vi "Teleop.vi"(10 "Match Info":T1={"Autonomous Elapsed Seconds"=0.0, "TeleOp Elapsed Seconds"=0.0, "Disabled Elapsed Seconds"=0.0, "Visited Autonomous"=FALSE, "Visited TeleOp"=FALSE, "Visited Disabled"=FALSE, "Autonomous Settings"={"Autonomous Style"=enum."Independent", "VI Refnum"=refnum}}, 11 "Call Context":T2) -> ()   [LabVIEW 2018]
doc: "This VI is called for each TeleOp packet received from the DS where the robot is not disabled. It is often used to read from the joysticks and update I/O or to update setpoints for timed control loops. It should complete and return within 20 milliseconds or it may miss DS packets."
uses:
  <vilib>/Rock Robotics/WPI/DriverStation/WPI_DriverStationDerivedRobotMode.ctl
  <vilib>/Rock Robotics/WPI/DriverStation/WPI_DriverStationMatch Info.ctl
  Functions/Global Variables/Robot State.vi
  Functions/Global Variables/Trajectory Enabled.vi
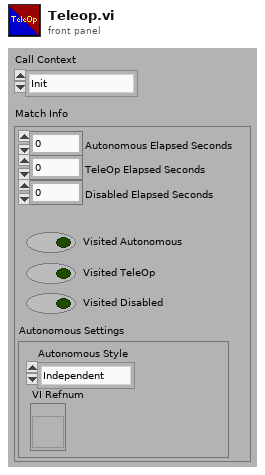
[diagram p1: front panel]
types:
  T1 = typedef "WPI_DriverStationMatch Info.ctl" = cluster{"Autonomous Elapsed Seconds":dbl, "TeleOp Elapsed Seconds":dbl, "Disabled Elapsed Seconds":dbl, "Visited Autonomous":bool, "Visited TeleOp":bool, "Visited Disabled":bool, "Autonomous Settings":cluster{"Autonomous Style":enum16{"Iterative", "Independent"}, "VI Refnum":refnum<vi>}}
  T2 = typedef "WPI_DriverStationDerivedRobotMode.ctl" = enum16{"Init", "Execute", "Stop"}
  T3 = typedef "Robot State.ctl" = cluster{"Drive System State":T4, "Climb System State":T7, "Arm System State":T8, "Ball System State":T9, "Disc System State":T10, "Lift System State":T11, "Grip System State":T12, "Enable Actions":T13}
  T4 = typedef "Robot Pivot Motion Commands.ctl" = cluster{"Front Right":T5, "Front Left":T5, "Rear Left":T5, "Rear Right":T5, "Drive Mode":T6}
  T5 = typedef "Pivot Motor Commands.ctl" = cluster{"Drive Power":dbl, "Drive Distance (in)":dbl, "Drive Distance Error (in)":dbl, "Steer Power":dbl, "Steer Angle (deg)":dbl, "Steer Angle Error (deg)":dbl}
  T6 = typedef "Robot Drive Mode.ctl" = enum16{"Velocity", "Distance"}
  T7 = typedef "Climb Motor Commands.ctl" = cluster{"Right Motor Power":dbl, "Right Motor Angle (deg)":dbl, "Right Motor Angle Error (deg)":dbl, "Left Motor Power":dbl, "Left Motor Angle (deg)":dbl, "Left Motor Angle Error (deg)":dbl}
  T8 = typedef "Arm Motor Commands.ctl" = cluster{"Enable Shoulder":bool, "Enable Elbow":bool, "Elbow Motor Power":dbl, "Sholder Motor Velocity":dbl}
  T9 = typedef "Ball Motor Commands.ctl" = cluster{"Intake Ball":bool, "Expel Ball":bool}
  T10 = typedef "Dics Eject Command.ctl" = cluster{"Eject Disk":bool}
  T11 = typedef "Lift Motor Commands.ctl" = cluster{"Lift Motor Power":dbl}
  T12 = typedef "Grip Motor Commands.ctl" = cluster{"Open Grip":bool, "Close Grip":bool}
  T13 = typedef "Enable Actions.ctl" = cluster{"Swerve Drive":bool, "Climber":bool, "Arm":bool, "Ball Intake":bool, "Disc Eject":bool, "Gripper":bool, "Lift":bool}
  T14 = typedef "DriveJoystickButtonMapping.ctl" = cluster{"relative encoders?":bool, "zero relative encoder":bool, "reset field orientation":bool, "use field orientation":bool, "braking":bool, "lock rotation":bool, "precision moves":bool}
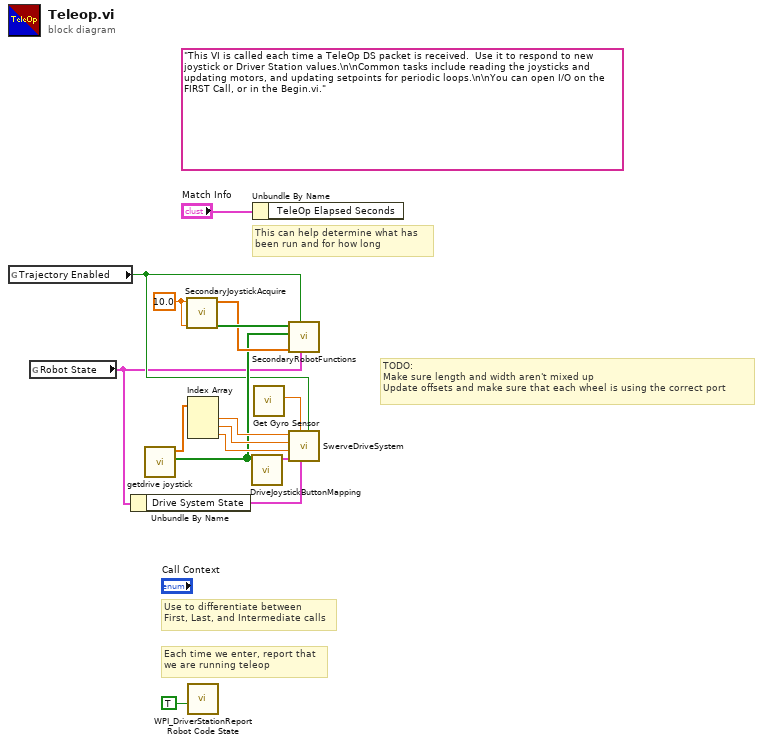
[diagram p0: block diagram]
diagram:
  w11 = 10.0 ("XY Joystick Deadband %")
  (unwired) "This VI is called each time a TeleOp DS packet is received.  Use it to respond to new joystick or Driver Station values.\n\nCommon tasks include reading the joysticks and updating motors, and updating setpoints for periodic loops.\n\nYou can open I/O on the FIRST Call, or in the Begin.vi."
  # "TODO:\nMake sure length and width aren't mixed up\nUpdate offsets and make sure that each wheel is using the correct port"
  # "Each time we enter, report that\nwe are running teleop"
  # "Use to differentiate between\nFirst, Last, and Intermediate calls"
  # "This can help determine what has\nbeen run and for how long"
  n1 = global read "Trajectory Enabled.vi" "Trajectory Enabled"() -> (w3:bool)
  n2 = global read "Robot State.vi" "Robot State"() -> (w2:T3)
  n3 = Unbundle By Name(w2) -> ("Drive System State"=w1:T4)
  n4 = call "getdrive joystick.vi"() -> ("drive joystick buttons"=w4:bool[], "drive joystick values"=w8:dbl[])  [unwired: 10 in]
  n5 = call "SecondaryJoystickAcquire.vi"("Rotation Joystick Deadband %"=w11, "XY Joystick Deadband %"=w11) -> ("Secondary Joystick Buttons"=w13:bool[], "Secondary Joystick Values"=w12:dbl[])  [unwired: 8 in]
  n6 = Index Array(array=w8) -> (element #1=w7:dbl, element #2=w6:dbl, element #3=w5:dbl)  [unwired: 3 in]
  n7 = call <vilib>:"WPI_DriverStationReport Robot Code State.vi"("TeleOp"=TRUE ("Autonomous")) -> ()  [unwired: 10 in, 1 out]
  n8 = call "DriveJoystickButtonMapping.vi"("drive joystick buttons"=w4) -> ("output cluster"=w9:T14)  [unwired: 9 in, 1 out]
  n9 = Unbundle By Name("Match Info") -> ()  [unwired: 1 out]
  n10 = call "Get Gyro Sensor.vi"() -> ("Robot Field Orientation (deg)"=w10:dbl)  [unwired: 11 in]
  n11 = call "SecondaryRobotFunctions.vi"("Robot State"=w2, "Automatic State Control Mode (F)"=w3, "Secondary Joystick Values"=w12, "Drive Joystick Buttons"=w4, "Secondary Joystick Buttons"=w13) -> ()  [unwired: 7 in]
  n12 = call "SwerveDriveSystem.vi"("Automatic State Control Mode (F)"=w3, "Robot Motion Commands"=w1, "Robot field orientation (deg)"=w10, "Drive Joystick Buttons"=w9, "Turn"=w5, "Forward"=w6, "Right"=w7) -> ()  [unwired: 5 in]
